vi "模擬缺點.vi"() -> ()   [LabVIEW 2015]
panel:
  in  "刪除點數":i32=10
  out "Image":T1(plugin-control)
  in  "Option":T2={"X個數"=20, "Y個數"=10, "起始X"=0.0, "起始Y"=0.0, "位移X"=20.0, "位移Y"=20.0, "抖動range"=0.0}
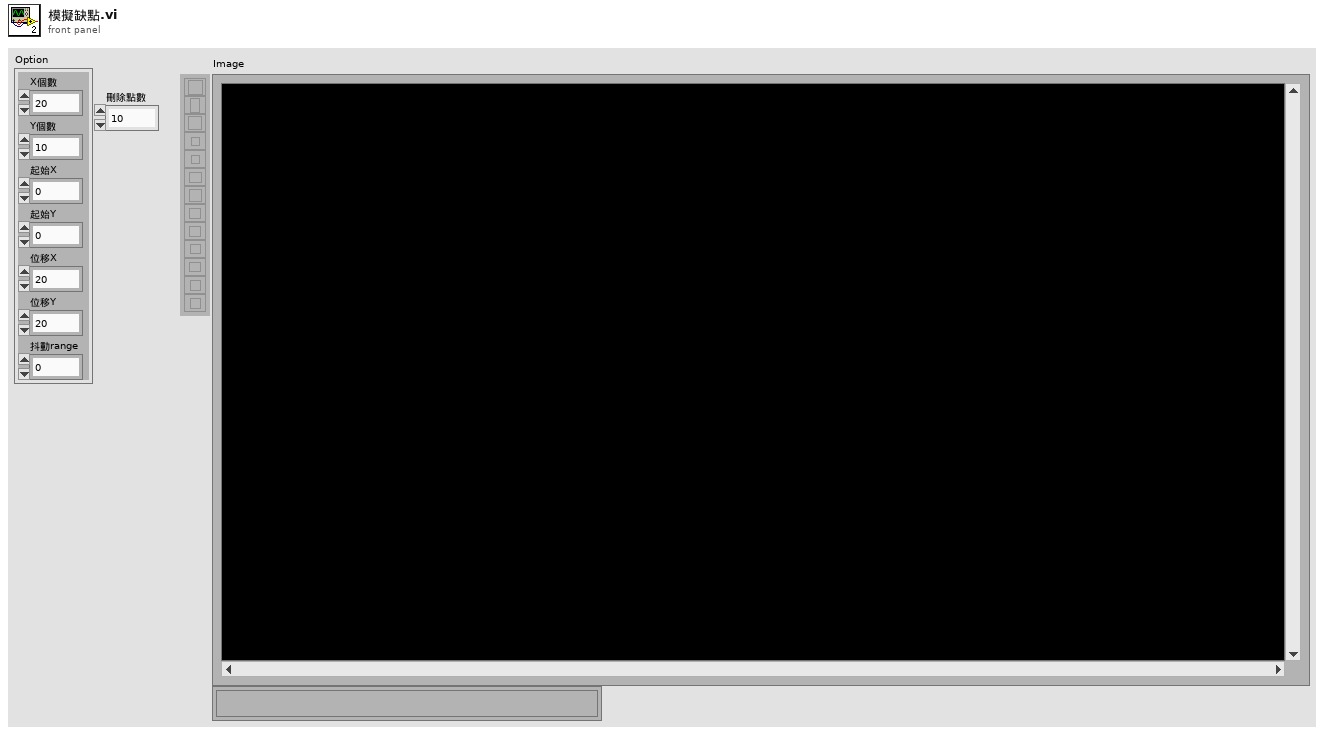
[diagram p1: front panel]
types:
  T1 = typedef "IMAQ Image.ctl" = refnum<image>
  T2 = cluster{"X個數":i32, "Y個數":i32, "起始X":dbl, "起始Y":dbl, "位移X":dbl, "位移Y":dbl, "抖動range":dbl}
  T3 = typedef "Image Type" = u32
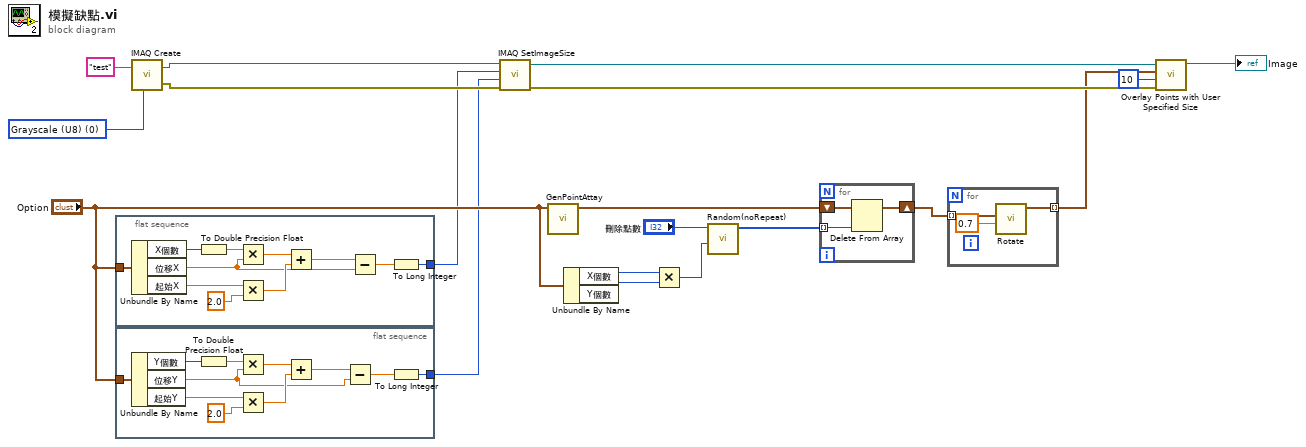
[diagram p0: block diagram]
diagram:
  w18 = T3 0 items=["Grayscale (U8)", "Grayscale (I16)", "Grayscale (SGL)", "Complex (CSG)", "RGB (U32)", "HSL (U32)", "RGB (U64)", "Grayscale (U16)"] ("Image Type")
  n1 = flat-sequence {
    tunnel: "Option" -> [w30]
    tunnel: [w20] -> w4
    frame #0 {
      n2 = Unbundle By Name(w30) -> ("X個數"=w29:i32, "位移X"=w22:dbl, "起始X"=w27:dbl)
      n3 = To Double Precision Float(number=w29) -> (double precision float=w28:dbl)
      n4 = Multiply(x=w28, y=w22) -> (x*y=w25:dbl)
      n5 = Multiply(x=w27, y=2.0) -> (x*y=w24:dbl)
      n6 = Add(x=w25, y=w24) -> (x+y=w23:dbl)
      n7 = Subtract(x=w23, y=w22) -> (x-y=w21:dbl)
      n8 = To Long Integer(number=w21) -> (32bit integer=w20:i32)
    }
  }
  n9 = flat-sequence {
    tunnel: "Option" -> [w41]
    tunnel: [w31] -> w3
    frame #0 {
      n10 = Unbundle By Name(w41) -> ("Y個數"=w40:i32, "位移Y"=w33:dbl, "起始Y"=w38:dbl)
      n11 = To Double Precision Float(number=w40) -> (double precision float=w39:dbl)
      n12 = Multiply(x=w39, y=w33) -> (x*y=w35:dbl)
      n13 = Multiply(x=w38, y=2.0) -> (x*y=w36:dbl)
      n14 = Add(x=w35, y=w36) -> (x+y=w34:dbl)
      n15 = Subtract(x=w34, y=w33) -> (x-y=w32:dbl)
      n16 = To Long Integer(number=w32) -> (32bit integer=w31:i32)
    }
  }
  n17 = call "IMAQ Create"("Image Name"="test", "Image Type"=w18) -> ("New Image"=w17:T1, "error out"=w16:errorcluster)  [unwired: 3 in]
  n18 = call "IMAQ SetImageSize"("error in (no error)"=w16, "Y Resolution"=w3, "X Resolution"=w4, "Image"=w17) -> ("error out"=w6:errorcluster, "Image Out"=w7:T1)  [unwired: 1 in]
  n19 = call <userlib>:"GenPointAttay.vi"("Option"="Option") -> ("Output Points"=w14:cluster{"X":dbl, "Y":dbl}[])  [unwired: 9 in, 1 out]
  n20 = Unbundle By Name("Option") -> ("X個數"=w13:i32, "Y個數"=w12:i32)
  n21 = Multiply(x=w13, y=w12) -> (x*y=w9:i32)
  n22 = call <userlib>:"Random(noRepeat).vi"("Max"=w9, "輸入點數"="刪除點數") -> ("Array"=w8:i32[])  [unwired: 9 in]
  n23 = for {
    tunnel: w8 -> [w42] mode=indexing
    shift-right: [w43] -> w2
    shift-left: w14 -> [w44]
    n24 = Delete From Array(array=w44, index=w42) -> (array with subset deleted=w43:cluster{"X":dbl, "Y":dbl}[])  [unwired: 1 in, 1 out]
  }
  n25 = for {
    tunnel: w2 -> [w47] mode=indexing
    tunnel: [w46] -> w1 mode=indexing
    n26 = call <userlib>:"Rotate.vi"("Rotate"=0.7, "Input Point"=w47) -> ("Output Point"=w46:cluster{"X":dbl, "Y":dbl})  [unwired: 8 in, 1 out]
  }
  n27 = call <userlib>:"Overlay Points with User Specified Size.vi"("error in"=w6, "Point Diameter (5)"=u32 10, "Points"=w1, "Image In"=w7) -> ("Image Out"=→"Image":T1)  [unwired: 6 in, 1 out]
